vi "Release-status-notifs.vi"(8 "error in (no error)":errorcluster, 11 "Object ref in":T1) -> (0 "error out":errorcluster, 3 "Object ref out":T1)   [LabVIEW 2013, in "HardwareCharacterization.lvlib" / "HC-Main.lvclass"]
uses:
  HC-Main.lvclass
  Object-reference.ctl
  HC-Main.lvclass/HC-Main.ctl
  Read Exit.vi
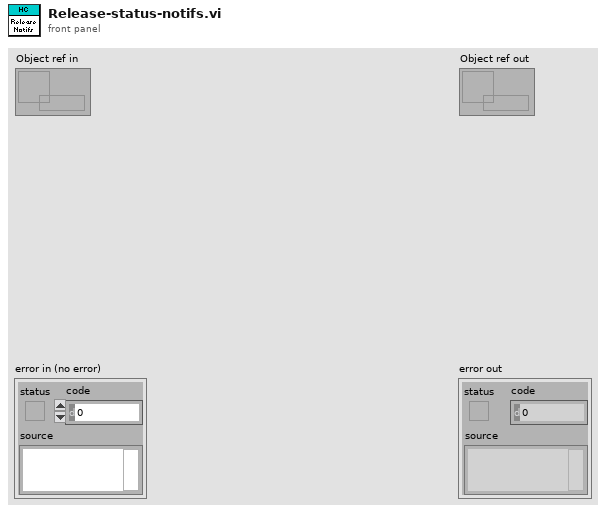
[diagram p1: front panel]
types:
  T1 = typedef "HardwareCharacterization.lvlib/HC-Main.lvclass/Object-reference.ctl" = refnum<data-value>
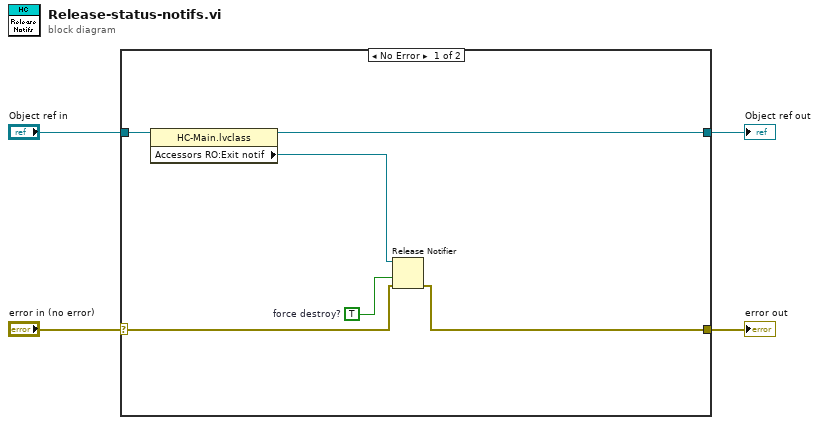
[diagram p0: block diagram]
diagram:
  n1 = case shown="No Error" "error in (no error)" {
    selector: "error in (no error)" -> [w7 w12]
    tunnel: [w5 w12] -> w3
    tunnel: [w9 w11] -> w1
    tunnel: "Object ref in" -> [w10 w11]
    frame No Error {
      w6 = TRUE  # force destroy?
      n2 = property class="HC-Main.lvclass"(reference=w10) -> (reference out=w9:T1, "Accessors RO:Exit notif"=w8:refnum<notifier>)  [unwired: 1 in, 1 out]
      n3 = Release Notifier(notifier=w8, force destroy? (F)=w6, error in (no error)=w7) -> (error out=w5:errorcluster)  [unwired: 2 out]
    }
    frame Error {
    }
  }
  "error out" <- w3
  "Object ref out" <- w1
